vi "SR1.constructor.vi"(0 "name":string, 2 "data in":string, 5 "error in (no error)":errorcluster) -> (14 "i ref out":refnum<vi>, 16 "data out":string, 19 "error out":errorcluster)   [LabVIEW 2014, in "SR1.lvlib"]
doc: "This is the constructor of a class.\n\nLicense Agreement for this software:\n\nCopyright (C)\nGesellschaft für Schwerionenforschung, GSI\nPlanckstr. 1\n64291 Darmstadt\nGermany\n\nContact: D.Beck@gsi.de \n\nThis program is free software; you can redistribute it and/or modify it under the terms of the \nGNU General Public License as published by the Free Software Foundation; either version 2 of \nthe license, or (at your option) any later version.\n\nThis program is distributed in the hope that it will be useful, but WITHOUT ANY WARRANTY; \nwithout even the implied warranty of MERCHANTABILITY or FITNESS FOR A PARTICULAR PURPOSE. See the GNU General License for more details (http://www.gnu.org).\n\nGesellschaft für Schwerionenforschung, GSI\nPlanckstr. 1, 64291 Darmstadt, Germany\nFor all questions and ideas contact: M.Richter@gsi.de, H.Brand@gsi.de or D.Beck@gsi.de.\nLast update: 16-JUN-2004"
uses:
  SR1.lvlib
  CS_Core/CSApplicationBaseClasses/DeviceBase/DeviceBase.myEventNames.ctl
  CS_Core/CSApplicationBaseClasses/NABase/NABase.myEventNames.ctl
  CS_Core/CSSystem/CSSystemLib/CSSystemLib.lvlib
  CS_Core/CSApplicationBaseClasses/DeviceBase/DeviceBase.lvlib
  CS_Core/CSApplicationBaseClasses/NABase/NABase.lvlib
  instr.lib/Stanford Research SR1/Stanford Research SR1.lvlib
  CS_Core/BaseProcess/BaseProcess.lvlib
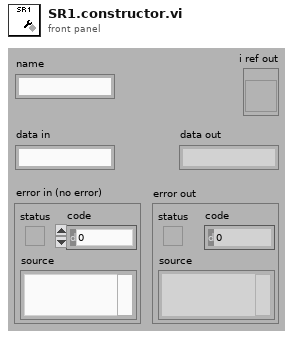
[diagram p1: front panel]
types:
  T1 = enum16{"SetAttribute", "GetAttribute", "CreateAttribute", "DestroyAttribute", "DestroyAllAtributes"}
  T2 = typedef "NABase.lvlib/NABase.myEventNames.ctl" = enum16{"lvmsg://SetStartFreq", "lvmsg://SetNofLines", "lvmsg://SetfreqSpan", "lvmsg://StartScan", "lvmsg://StopScan", "lvmsg://GetScanStatus", "lvmsg://GetData", "lvmsg://GetStartFreq", "lvmsg://GetNofLines", "lvmsg://GetFreqSpan", "lvmsg://SetTriggerLevel", "lvmsg://SetTriggerSlope", "lvmsg://GetTriggerLevel", "lvmsg://GetTriggerSlope", "lvmsg://ReadData", "lvmsg://GetTimeRecDur", "lvmsg://GetNofStoredData"}
  T3 = typedef "DeviceBase.lvlib/DeviceBase.myEventNames.ctl" = enum16{"lvmsg://Initialize", "lvmsg://Close", "lvmsg://Configure", "lvmsg://Reset", "lvmsg://IDQuery"}
  T4 = typedef "BaseProcess.lvlib/BaseProcess.i attribute.ctl" = cluster{"EventStatus":string, "EventError":i32, "PresetEvtWatchD":i32, "PresetPdcWatchD":i32, "EventTimeout":i32, "PeriodicInterval":i32, "Interface":string[], "Address":string[], "Special":string[], "PeriodicError":i32, "PeriodicStatus":string, "SuperProc":string, "Descriptors":T5[], "CaseRef":refnum<vi>, "PdcRef":refnum<vi>, "Thread Ref":refnum<vi>, "eventErrorID":i32, "eventStatusID":i32, "periodicErrorID":i32, "periodicStatusID":i32, "pdcCtrID":i32}
  T5 = typedef "BaseProcess.lvlib/BaseProcess.descriptor definition.ctl" = cluster{"selector":string, "descriptor":T6}
  T6 = typedef "BaseProcess.lvlib/BaseProcess.descriptor string definition.ctl" = string
  T7 = typedef "SR1.lvlib/SR1.i attribute.ctl" = cluster{"GraphID":i32, "TraceID":i32, "MaxWait":i32}
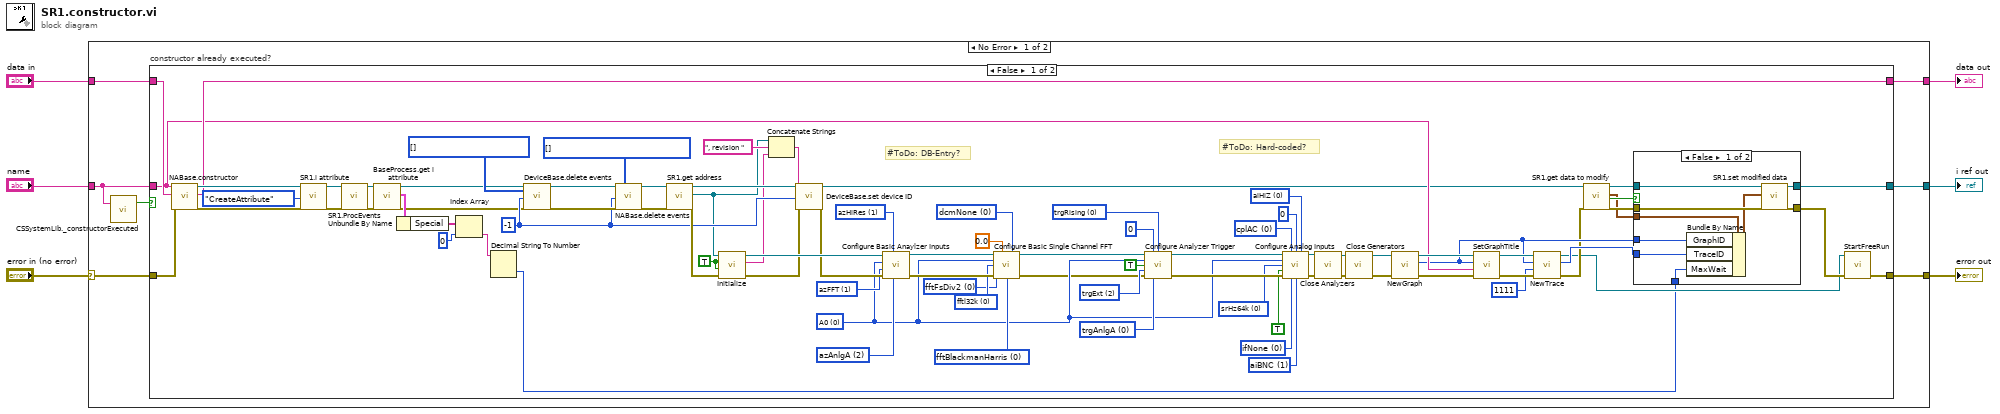
[diagram p0: block diagram]
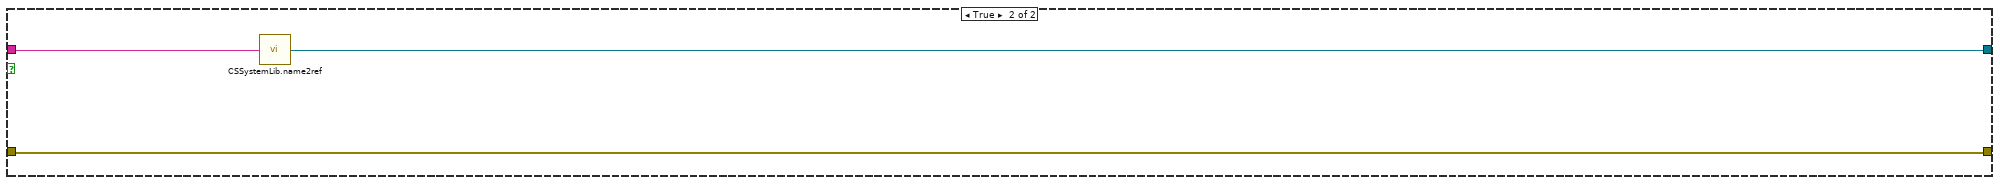
[diagram p3: hidden frame]
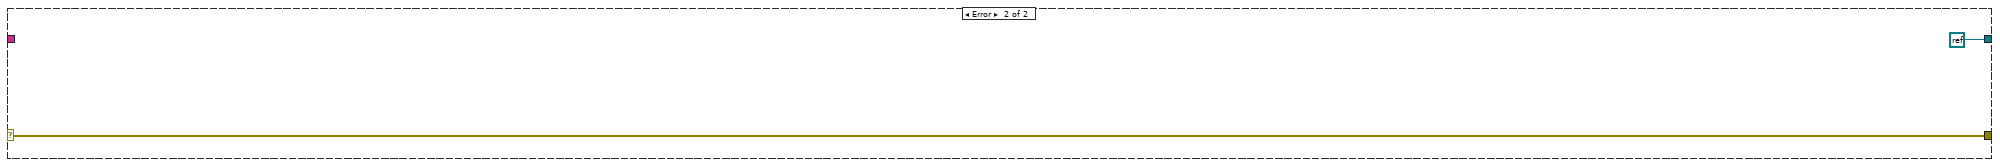
[diagram p4: hidden frame]
diagram:
  n1 = case shown="No Error" "error in (no error)" {
    selector: "error in (no error)" -> [w11 w113]
    tunnel: "name" -> [w10 _]
    tunnel: [w13 refnum<k0> refnum ("Not a Refnum Constant")] -> w5
    tunnel: [w12 w113] -> w4
    tunnel: "data in" -> [w8 _]
    tunnel: [w7 _] -> w1
    frame No Error {
      n2 = call "CSSystemLib._constructorExecuted.vi"("name"=w10) -> ("constructor executed?"=w9:bool)  [unwired: 18 in]
      n3 = case "constructor already executed?" shown="False" w9 {
        tunnel: w10 -> [w67 w112]
        tunnel: [w65 w111] -> w13
        tunnel: [w25 w110] -> w12
        tunnel: w11 -> [w93 w110]
        tunnel: w8 -> [w92 _]
        tunnel: [w88 _] -> w7
        frame False {
          w27 = T2[] [] items=["lvmsg://SetStartFreq", "lvmsg://SetNofLines", "lvmsg://SetfreqSpan", "lvmsg://StartScan", "lvmsg://StopScan", "lvmsg://GetScanStatus", "lvmsg://GetData", "lvmsg://GetStartFreq", "lvmsg://GetNofLines", "lvmsg://GetFreqSpan", "lvmsg://SetTriggerLevel", "lvmsg://SetTriggerSlope", "lvmsg://GetTriggerLevel", "lvmsg://GetTriggerSlope", "lvmsg://ReadData", "lvmsg://GetTimeRecDur", "lvmsg://GetNofStoredData"] ("events")
          w32 = 0 items=["srHz64k", "srHz128k", "srOSR", "srOSRx2"] ("Hi-Res Sample Rate (0: srHz64k)")
          w34 = 1 items=["aiXLR", "aiBNC", "aiGenMon", "aiDigCommonMode"] ("Source (0: aiXLR)")
          w35 = 0 items=["ifNone", "ifFiler1", "ifFilter2", "ifFilter3", "ifFilter4", "ifGround"] ("Optional Filter (0: ifNone)")
          w36 = u16 0 items=["cplAC", "cplDC"] ("Coupling (0: cplAC)")
          w38 = 0 items=["aiHiZ", "aiz300", "aiz600"] ("Zin (0: aiHiZ)")
          w39 = 0 items=["trgAnlgA", "trgAnlgB", "trgDigA", "trgDigB", "trgJitter"] ("Generator Trigger Source (0: trgAnlgA)")
          w40 = 2 items=["trgInputCh", "trgOtherCh", "trgExt", "trgManual", "trgGen", "trgDigAudBlock", "trgBurstA", "trgBurstB"] ("Trigger Source (0: trgInputCh)")
          w28 = u16 0 items=["trgRising", "trgFalling"] ("Trigger Polarity (0: trgRising)")
          w43 = 0 items=["fftFsDiv2", "fftFsDiv4", "fftFsDiv8", "fftFsDiv16", "fftFsDiv32", "fftFsDiv64", "fftFsDiv128", "fftFsDiv256", "fftFsDiv512", "fftFsDiv1024"] ("Frequency Span (0: fftFsDiv2)")
          w44 = 0 items=["fftl32k", "fftl16k", "fftl8k", "fftl4k", "fftl2k", "fftl1k", "fftl512", "fftl256"] ("Lines (0: fftl32k)")
          w45 = 0 items=["fftBlackmanHarris", "fftHann", "fftHamming", "fftEquiripple", "fftFlattop", "fftGaussian", "fftKaiser", "fftUniform", "fftRifeVincent4", "fftRifeVincent5", "fftRifeVincent10", "fftBlackmanHarris7", "fftVariable"] ("FFT Window (0: fftBlackmanHarris)")
          w47 = 0 items=["dcmNone", "dcmMean", "dcmPkPK"] ("DC Correction Mode (0: dcmNone)")
          w48 = 2 items=["azAnlg", "azDig", "azAnlgA", "azAnlgB", "azDigA", "azDigB", "azDetOut"] ("Input Source (0: azAnlg)")
          w49 = 1 items=["azTimeDomeDet", "azFFT", "azFFT2Ch", "azTHD", "azIMD", "azMultitone", "azJitter", "azHistogram", "azOctave"] ("Measurement Function (0: azTimeDomeDet)")
          w31 = 0 items=["A0", "A1"] ("Analyzer (0: A0)")
          w50 = 1 items=["azHiBW", "azHiRes", "azISR", "azDetOutSR"] ("Sample Rate (0: azHiBW)")
          w84 = TRUE ("ID Query (True)")
          w91 = T3[] [] items=["lvmsg://Initialize", "lvmsg://Close", "lvmsg://Configure", "lvmsg://Reset", "lvmsg://IDQuery"] ("events")
          w53 = -1 ("ms timeout (10000)")
          # "#ToDo: Hard-coded?"
          # "#ToDo: DB-Entry?"
          n4 = call "NABase.constructor.vi"("name"=w67, "data in"=w92, "error in (no error)"=w93) -> ("i ref out"=w98:refnum<vi>, "data out"=w88:string, "error out"=w97:errorcluster)  [unwired: 14 in]
          n5 = call "SR1.i attribute.vi"("VI Refnum"=w98, "Action"=T1."CreateAttribute", "error in (no error)"=w97) -> ("VI Refnum out"=w95:refnum<vi>, "error out"=w94:errorcluster)  [unwired: 14 in, 1 out]
          n6 = call "SR1.ProcEvents.vi"("i ref in"=w95, "error in (no error)"=w94) -> ("i ref out"=w20:refnum<vi>, "error out"=w21:errorcluster)  [unwired: 16 in]
          n7 = call "BaseProcess.get i attribute.vi"("i ref in"=w20, "error in (no error)"=w21) -> ("i ref out"=w19:refnum<vi>, "i attribute"=w22:T4, "error out"=w18:errorcluster)  [unwired: 15 in]
          n8 = Unbundle By Name(w22) -> ("Special"=w17:string[])
          n9 = Index Array(array=w17, index=0 ("Index")) -> (element=w15:string)
          n10 = Decimal String To Number(string=w15) -> (number=w14:i32)  [unwired: 2 in, 1 out]
          n11 = call "DeviceBase.delete events.vi"("i ref in"=w19, "events"=w91, "ms timeout (10000)"=w53, "error in (no error)"=w18) -> ("i ref out"=w90:refnum<vi>, "error out"=w89:errorcluster)  [unwired: 13 in, 1 out]
          n12 = call "NABase.delete events.vi"("i ref in"=w90, "events"=w27, "ms timeout (10000)"=w53, "error in (no error)"=w89) -> ("i ref out"=w86:refnum<vi>, "error out"=w87:errorcluster)  [unwired: 13 in, 1 out]
          n13 = call "SR1.get address.vi"("i ref in"=w86, "error in (no error)"=w87) -> ("i ref out"=w56:refnum<vi>, "VISA resource name"=w51:refnum<visa-resource-name>, "error out"=w85:errorcluster)  [unwired: 15 in]
          n14 = call "Initialize.vi"("error in (no error)"=w85, "Reset (True)"=w84, "ID Query (True)"=w84, "VISA resource name"=w51) -> ("error out"=w55:errorcluster, "ID"=w52:string, "VISA resource name out"=w83:refnum<visa-resource-name>)  [unwired: 5 in]
          n15 = Concatenate Strings(w51, ", revision " ("string"), w52) -> (w57:string)
          n16 = call "DeviceBase.set device ID.vi"("i ref in"=w56, "deviceID"=w57, "ms timeout (10000)"=w53, "error in (no error)"=w55) -> ("i ref out"=w30:refnum<vi>, "error out"=w54:errorcluster)  [unwired: 13 in, 1 out]
          n17 = call "Configure Basic Anaylzer Inputs.vi"("Input Source (0: azAnlg)"=w48, "Sample Rate (0: azHiBW)"=w50, "error in (no error)"=w54, "Measurement Function (0: azTimeDomeDet)"=w49, "Analyzer (0: A0)"=w31, "VISA resource name"=w83) -> ("error out"=w81:errorcluster, "VISA resource name out"=w82:refnum<visa-resource-name>)  [unwired: 4 in]
          n18 = call "Configure Basic Single Channel FFT .vi"("VISA resource name"=w82, "Start Frequency (0 mHz)"=0.0 ("Stop Frequency (0 mHz)"), "DC Correction Mode (0: dcmNone)"=w47, "Analyzer (0: A0)"=w31, "Lines (0: fftl32k)"=w44, "Frequency Span (0: fftFsDiv2)"=w43, "error in (no error)"=w81, "FFT Window (0: fftBlackmanHarris)"=w45) -> ("VISA resource name out"=w80:refnum<visa-resource-name>, "error out"=w29:errorcluster)  [unwired: 6 in]
          n19 = call "Configure Analyzer Trigger.vi"("VISA resource name"=w80, "Jitter Level (0 %FS)"=0, "Trigger Polarity (0: trgRising)"=w28, "Analyzer (0: A0)"=w31, "Enable Trigger (T: Enable)"=TRUE, "Trigger Source (0: trgInputCh)"=w40, "error in (no error)"=w29, "Generator Trigger Source (0: trgAnlgA)"=w39) -> ("VISA resource name out"=w78:refnum<visa-resource-name>, "error out"=w79:errorcluster)  [unwired: 6 in]
          n20 = call "Configure Analog Inputs.vi"("VISA resource name"=w78, "Coupling (0: cplAC)"=w36, "Range (0)"=0, "Zin (0: aiHiZ)"=w38, "Channel (0: ChannelA)"=w31, "Hi-Res Sample Rate (0: srHz64k)"=w32, "Auto Range (T: Enable)"=TRUE, "error in (no error)"=w79, "Optional Filter (0: ifNone)"=w35, "Source (0: aiXLR)"=w34) -> ("VISA resource name out"=w74:refnum<visa-resource-name>, "error out"=w75:errorcluster)  [unwired: 4 in]
          n21 = call "Close Analyzers.vi"("error in (no error)"=w75, "VISA resource name"=w74) -> ("error out"=w77:errorcluster, "VISA resource name out"=w76:refnum<visa-resource-name>)  [unwired: 8 in]
          n22 = call "Close Generators.vi"("error in (no error)"=w77, "VISA resource name"=w76) -> ("error out"=w72:errorcluster, "VISA resource name out"=w73:refnum<visa-resource-name>)  [unwired: 8 in]
          n23 = call "NewGraph.vi"("error in (no error)"=w72, "VISA resource name"=w73) -> ("error out"=w70:errorcluster, "GraphID"=w61:i32, "VISA resource name out"=w69:refnum<visa-resource-name>)  [unwired: 7 in]
          n24 = call "SetGraphTitle.vi"("error in (no error)"=w70, "Title"=w67, "GraphID"=w61, "VISA resource name"=w69) -> ("error out"=w71:errorcluster, "VISA resource name out"=w68:refnum<visa-resource-name>)  [unwired: 6 in]
          n25 = call "NewTrace.vi"("error in (no error)"=w71, "TraceType"=1111, "GraphID"=w61, "VISA resource name"=w68) -> ("error out"=w26:errorcluster, "TraceID"=w60:i32, "VISA resource name out"=w23:refnum<visa-resource-name>)  [unwired: 5 in]
          n26 = call "SR1.get data to modify.vi"("i ref in"=w30, "error in (no error)"=w26) -> ("i ref out"=w66:refnum<vi>, "i attribute"=w62:T7, "timed out"=w63:bool, "error out"=w64:errorcluster)  [unwired: 14 in]
          n27 = case shown="False" w63 {
            tunnel: w66 -> [w107 w109]
            tunnel: [w106 w109] -> w65
            tunnel: w64 -> [w105 w108]
            tunnel: [w104 w108] -> w24
            tunnel: w62 -> [w103 _]
            tunnel: w61 -> [w101 _]
            tunnel: w60 -> [w100 _]
            tunnel: w14 -> [w99 _]
            frame False {
              n28 = Bundle By Name(cluster=w103, "GraphID"=w101, "TraceID"=w100, "MaxWait"=w99) -> (w102:T7)
              n29 = call "SR1.set modified data.vi"("i ref in"=w107, "i attribute"=w102, "error in (no error)"=w105) -> ("i ref out"=w106:refnum<vi>, "error out"=w104:errorcluster)  [unwired: 15 in]
            }
            frame True {
            }
          }
          n30 = call "StartFreeRun.vi"("error in (no error)"=w24, "VISA resource name"=w23) -> ("error out"=w25:errorcluster)  [unwired: 8 in, 1 out]
        }
        frame True {
          n31 = call "CSSystemLib.name2ref.vi"("name"=w112) -> ("obj refnum"=w111:refnum<vi>)
        }
      }
    }
    frame Error {
    }
  }
  "i ref out" <- w5
  "error out" <- w4
  "data out" <- w1
